vi "Read Heartbeat interval.vi"(8 "error in (no error)":errorcluster, 11 "Client in":refnum<class "SC-Client.lvclass">) -> (0 "error out":errorcluster, 2 "Heartbeat interval":dbl format="%.2f", 3 "Client out":refnum<class "SC-Client.lvclass">)   [LabVIEW 2013, in "SLMControl.lvlib" / "SC-Client.lvclass"]
uses:
  SC-Client.lvclass
  SC-Client.lvclass/SC-Client.ctl
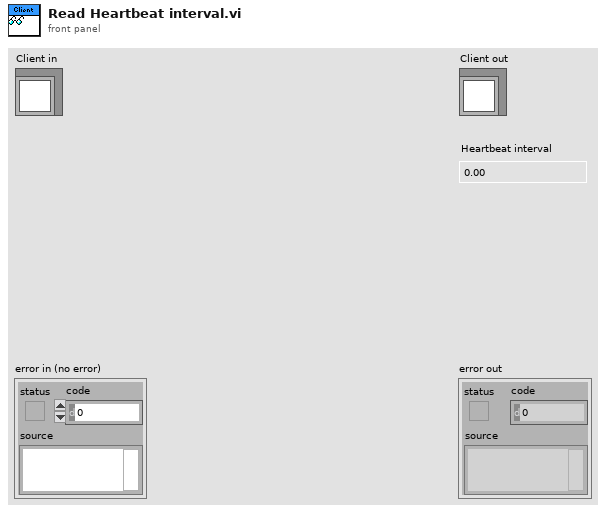
[diagram p1: front panel]
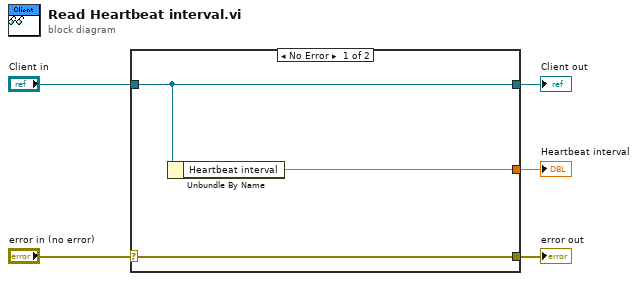
[diagram p0: block diagram]
diagram:
  n1 = case shown="No Error" "error in (no error)" {
    selector: "error in (no error)" -> [w8 w9]
    tunnel: [w8 w9] -> w4
    tunnel: [w7 w10] -> w2
    tunnel: "Client in" -> [w7 w10]
    tunnel: [w6 _] -> w1
    frame No Error {
      n2 = Unbundle By Name(w7) -> ("Heartbeat interval"=w6:dbl)
    }
    frame Error {
    }
  }
  "error out" <- w4
  "Client out" <- w2
  "Heartbeat interval" <- w1
